vi "SpectroMeterRead.vi"(2 "error IO":errorcluster caption="error in") -> (0 "error IO 2":errorcluster caption="error out")   [LabVIEW 2018]
panel:
  in  "停止":bool
  in  "开始测量":bool
  in  "更改参数":bool
  out "重频":dbl caption="重复频率" format="%.2f"
  out "脉宽":dbl caption="脉冲宽度" format="%.2f"
  out "时间波形":waveform(dbl)(graph)
  # "光   谱"
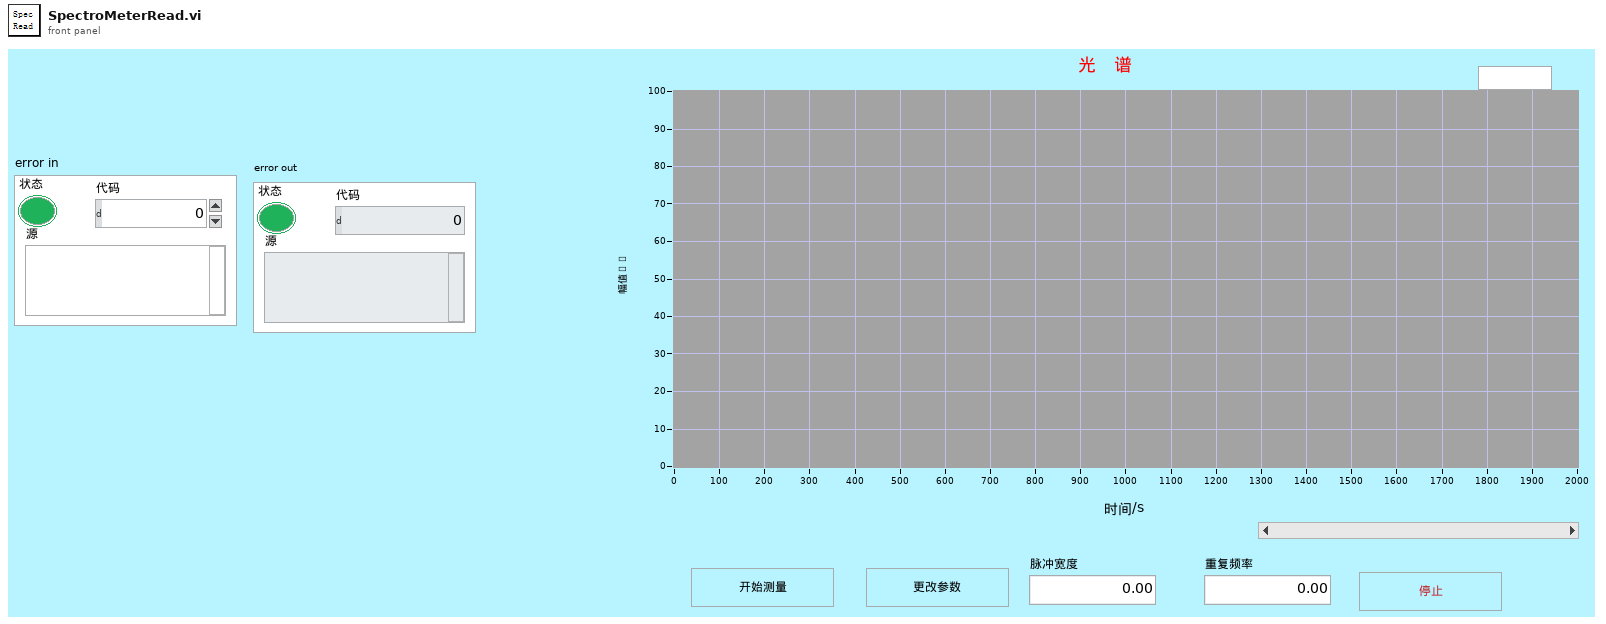
[diagram p1: front panel]
types:
  T1 = enum16{"功率测量", "能量测量", "光谱测量", "时间波形", "偏振测量", "近远场"}
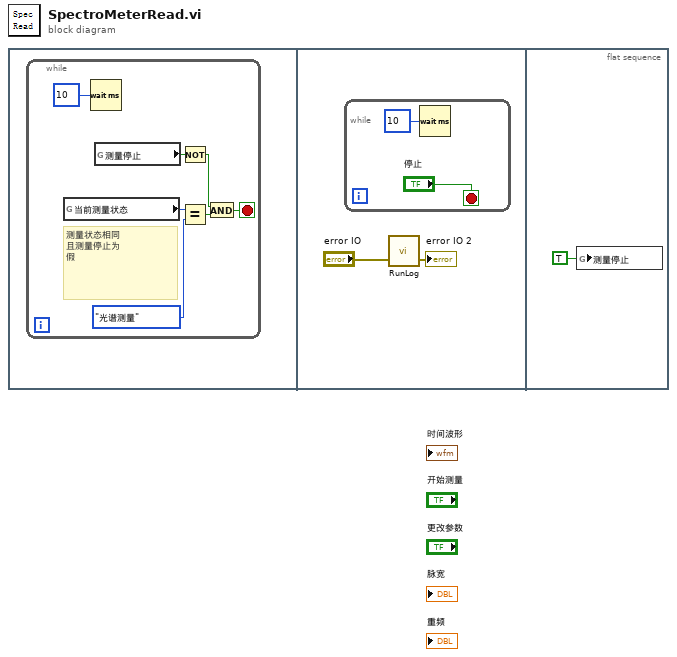
[diagram p0: block diagram]
diagram:
  n1 = flat-sequence {
    frame #0 {
      n2 = while {
        stop <- w4 stop-if-true
        # "测量状态相同\n且测量停止为\n假"
        n3 = global read "参数.vi" "当前测量状态"() -> (w2:T1)
        n4 = Wait (ms)(milliseconds to wait=u32 10 ("等待时间（毫秒）")) -> ()  [unwired: 1 out]
        n5 = global read "参数.vi" "测量停止"() -> (w5:bool)
        n6 = Not(x=w5) -> (.not. x?=w6:bool)
        n7 = Equal?(x=w2, y=T1."光谱测量" ("当前测量状态")) -> (x = y?=w1:bool)
        n8 = And(x=w6, y=w1) -> (x .and. y?=w4:bool)
      }
    }
    frame #1 {
      n9 = while {
        stop <- "停止" stop-if-true
        n10 = Wait (ms)(milliseconds to wait=u32 10 ("等待时间（毫秒）")) -> ()  [unwired: 1 out]
      }
      n11 = call "RunLog.vi"("error in"="error IO") -> ("error out"=→"error IO 2":errorcluster)  [unwired: 2 in]
    }
    frame #2 {
      n12 = global write "参数.vi" "测量停止"(TRUE ("测量停止")) -> ()
    }
  }
